vi "Actor Core.vi"(8 "error in":errorcluster, 11 "State in":refnum<class "State Machine.lvclass">) -> (0 "error out":errorcluster, 3 "Actor out":refnum<class "Actor.lvclass">)   [LabVIEW 2013, in "State Machine.lvclass"]
doc: "(<B>Filename</B>: Actor Framework.lvlib:Actor.lvclass:Actor Core.vi)\n\nThis override invokes Entry.vi on the initial state, prior to calling the parent Actor Core. Adding this behavior to Actor Core (instead of an override of Pre Launch Init.vi) allows the initial state to launch a nested actor as part of its entry behavior.\n\nReceives messages to the actor, reacts to them, and initiates any error handling that may shut the actor down.\n\nDescendant classes may override this VI to append parallel tasks for the actor to complete while it handles messages. Overrides use the Call Parent Method node."
uses:
  State Machine.lvclass
  <vilib>/ni/Actors/State Actor/State Actor/State Actor.lvclass
  <vilib>/ActorFramework/Actor/Actor.lvclass
panel:
  in  "Command State Status":T1
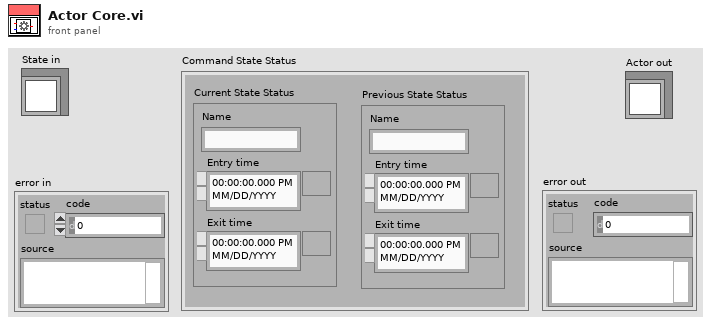
[diagram p1: front panel]
types:
  T1 = cluster{"Current State Status":cluster{"Name":string, "Entry time":timestamp, "Exit time":timestamp}, "Previous State Status":cluster{"Name":string, "Entry time":timestamp, "Exit time":timestamp}}
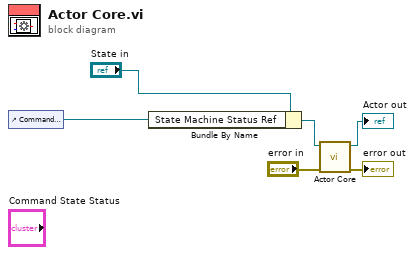
[diagram p0: block diagram]
diagram:
  n1 = control-ref of="Command State Status"() -> (w1:refnum<vi>)
  n2 = Bundle By Name(cluster="State in", "State Machine Status Ref"=w1) -> (w2:refnum<class "State Machine.lvclass">)
  n3 = call-parent "Actor Core.vi"("error in"="error in", "State in"=w2) -> ("error out"=→"error out":errorcluster, "Actor out"=→"Actor out":refnum<class "Actor.lvclass">)  [unwired: 8 in]
